vi "Agilent 34970 Channel Cycle.vi"(6 "Cycle Time (mS)":u32=1000, 8 "error in (no error)":errorcluster, 9 "Channel":string, 10 "Number Of Cycles":i32, 11 "VISA Refnum in":refnum<visa-resource-name>) -> (0 "error out":errorcluster, 3 "VISA Resource Name Out":refnum<visa-resource-name>)   [LabVIEW 2016]
uses:
  Agilent 34970.lvlib
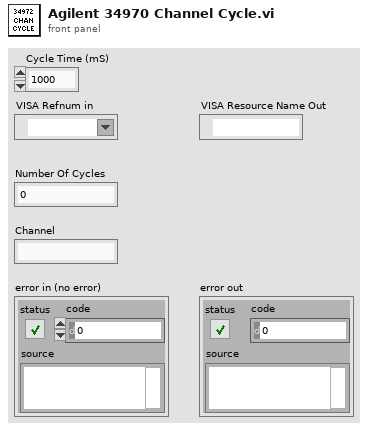
[diagram p1: front panel]
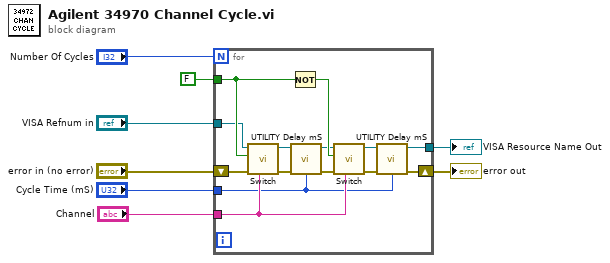
[diagram p0: block diagram]
diagram:
  n1 = for {
    N: "Number Of Cycles" -> [_]
    tunnel: "Channel" -> [w17]
    tunnel: "VISA Refnum in" -> [w11]
    shift-right: [w13] -> w6
    shift-left: "error in (no error)" -> [w15]
    tunnel: FALSE -> [w12]
    tunnel: "Cycle Time (mS)" -> [w10]
    tunnel: [w9] -> w1
    n2 = call "Switch.vi"("Channel List(empty)"=w17, "error in (no error)"=w15, "Open/Close (F:Close)"=w12, "VISA Resource Name"=w11) -> ("error out"=w19:errorcluster, "VISA Resource Name Out"=w16:refnum<visa-resource-name>)  [unwired: 5 in, 1 out]
    n3 = Not(x=w12) -> (.not. x?=w18:bool)
    n4 = call "UTILITY Delay mS.vi"("Error In"=w19, "milliseconds to wait"=w10) -> ("Error Out"=w20:errorcluster)  [unwired: 13 in]
    n5 = call "Switch.vi"("Channel List(empty)"=w17, "error in (no error)"=w20, "Open/Close (F:Close)"=w18, "VISA Resource Name"=w16) -> ("error out"=w14:errorcluster, "VISA Resource Name Out"=w9:refnum<visa-resource-name>)  [unwired: 5 in, 1 out]
    n6 = call "UTILITY Delay mS.vi"("Error In"=w14, "milliseconds to wait"=w10) -> ("Error Out"=w13:errorcluster)  [unwired: 13 in]
  }
  "error out" <- w6
  "VISA Resource Name Out" <- w1
